vi "LakeShore 340 Read.vi"(2 "Point #":i32, 3 "Parameters":dbl[](array[numeric]) format="%.3e", 4 "Instrument Address":refnum<visa-resource-name>) -> (0 "Stop":bool, 1 "Measurement":dbl[](array[numeric]) format="%.6e")   [LabVIEW 2025]
doc: "This VI reads a single reading from a LakeShore 340 Temperature Controller. The stop boolean is always false. If no reading is obtained a single zero is returned.\nParameter 0 - 0=Resistance, 1=Temperature, 2=Heater Power\nParameter 1 - Channel to read, channel 0 is channel A, etc.\nScott Hannahs, <sth@magnet.fsu.edu> NHMFL-FSU, May 2003\nAuthor: Scott Hannahs <sth@magnet.fsu.edu>\n\nThis software is licensed for use under the “MIT License\"\nCopyright (c) 2025 Scott Hannahs, sth@sth@magnet.sthnet.net\n\nPermission is hereby granted, free of charge, to any person obtaining a copy of this software and associated documentation files (the \"Software\"), to deal in the Software without restriction, including without limitation the rights to use, copy, modify, merge, publish, distribute, sublicense, and/or sell copies of the Software, and to permit persons to whom the Software is furnished to do so, subject to the following conditions: The above copyright notice and this permission notice shall be included in all copies or substantial portions of the Software.\n\nTHE SOFTWARE IS PROVIDED \"AS IS\", WITHOUT WARRANTY OF ANY KIND, EXPRESS OR IMPLIED, INCLUDING BUT NOT LIMITED TO THE WARRANTIES OF MERCHANTABILITY, FITNESS FOR A PARTICULAR PURPOSE AND NONINFRINGEMENT. IN NO EVENT SHALL THE AUTHORS OR COPYRIGHT HOLDERS BE LIABLE FOR ANY CLAIM, DAMAGES OR OTHER LIABILITY, WHETHER IN AN ACTION OF CONTRACT, TORT OR OTHERWISE, ARISING FROM, OUT OF OR IN CONNECTION WITH THE SOFTWARE OR THE USE OR OTHER DEALINGS IN THE SOFTWARE."
panel:
  # "The first parameter tells it\nHeater power if =2\nto read temperature if =1\nResistance if =0\nThe second is channel #"
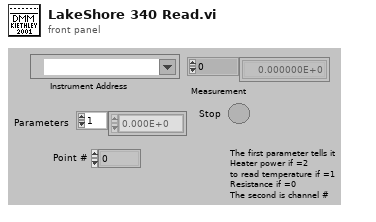
[diagram p1: front panel]
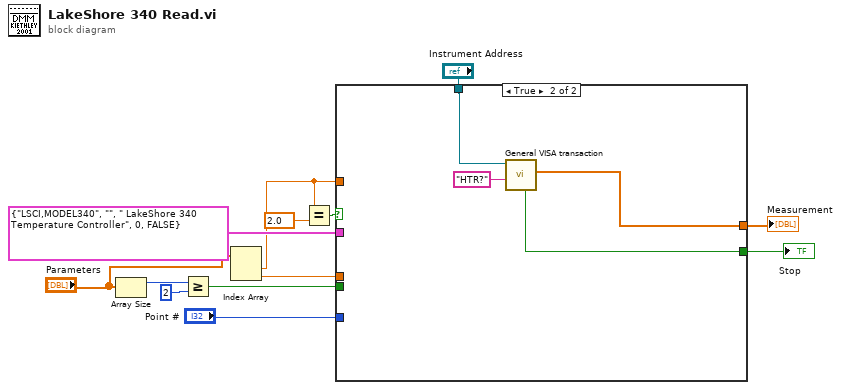
[diagram p0: block diagram]
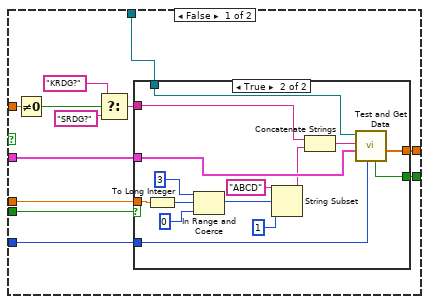
[diagram p2: hidden frame]
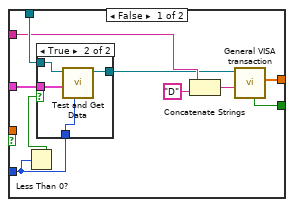
[diagram p3: hidden frame]
diagram:
  n1 = Array Size(array="Parameters") -> (size(s)=w7:i32)
  n2 = Greater Or Equal?(x=w7, y=2) -> (x >= y?=w10:bool)
  n3 = Index Array(array="Parameters") -> (element #1=w3:dbl, element #2=w5:dbl)  [unwired: 2 in]
  n4 = Equal?(x=w3, y=2.0) -> (x = y?=w4:bool)
  n5 = case shown="True" w4 {
    tunnel: cluster{string, string, string, u32, bool} {"LSCI,MODEL340", "", " LakeShore 340 Temperature Controller", 0, FALSE} -> [w25 _]
    tunnel: [w24 w57] -> w12
    tunnel: [w23 w56] -> w11
    tunnel: w10 -> [w22 _]
    tunnel: "Point #" -> [w21 _]
    tunnel: w5 -> [w20 _]
    tunnel: w3 -> [w19 _]
    tunnel: "Instrument Address" -> [w14 w59]
    frame False {
      n6 = Not Equal To 0?(x=w19) -> (x != 0?=w18:bool)
      n7 = Select(t="KRDG?" ("Format String"), s=w18, f="SRDG?" ("Format String")) -> (s? t:f=w17:string)
      n8 = case shown="True" w22 {
        tunnel: w25 -> [w35 w52]
        tunnel: w14 -> [w34 w55]
        tunnel: [w33 w51] -> w24
        tunnel: [w32 w50] -> w23
        tunnel: w21 -> [w30 w54]
        tunnel: w20 -> [_ w46]
        tunnel: w17 -> [w29 w45]
        frame False {
          n9 = Less Than 0?(x=w30) -> (x < 0?=w31:bool)
          n10 = case shown="True" w31 {
            tunnel: w35 -> [_ w40]
            tunnel: w34 -> [w36 w39]
            tunnel: w30 -> [_ w38]
            tunnel: [w36 w37] -> w26
            frame False {
            }
            frame True {
              n11 = call "Test and Get Data.vi"("Point #"=w38, "Instrument Info"=w40, "VISA Sesson"=w39) -> ("dup VISA session"=w37:refnum<visa-resource-name>)  [unwired: 3 in, 4 out]
            }
          }
          n12 = Concatenate Strings(w29, "D" ("string")) -> (w28:string)
          n13 = call "General VISA transaction.vi"("Command String"=w28, "VISA Session"=w26) -> ("Measurement"=w33:dbl[], "Stop"=w32:bool)  [unwired: 4 in, 4 out]
        }
        frame True {
          n14 = To Long Integer(number=w46) -> (32bit integer=w47:i32)
          n15 = In Range and Coerce(upper limit=3, x=w47, lower limit=0) -> (coerced(x)=w42:i32)  [unwired: 1 out]
          n16 = String Subset(string="ABCD", offset (0)=w42, length (rest)=1 ("length (rest)")) -> (substring=w41:string)
          n17 = Concatenate Strings(w45, w41) -> (w53:string)
          n18 = call "Test and Get Data.vi"("Point #"=w54, "Instrument Info"=w52, "Command String"=w53, "VISA Sesson"=w55) -> ("Measurement"=w51:dbl[], "Stop"=w50:bool)  [unwired: 2 in, 3 out]
        }
      }
    }
    frame True {
      n19 = call "General VISA transaction.vi"("Command String"="HTR?", "VISA Session"=w59) -> ("Measurement"=w57:dbl[], "Stop"=w56:bool)  [unwired: 4 in, 4 out]
    }
  }
  "Stop" <- w11
  "Measurement" <- w12
